vi "Lockin.vi"   [LabVIEW 2019, in "Instrument.Lockin.lvlib"]
uses:
  Instrument.Lockin.lvlib
  Instrument.Lockin/Instrument.Lockin.AppLauncher.vi
  Instrument.Lockin/Instrument.Lockin.lvclass
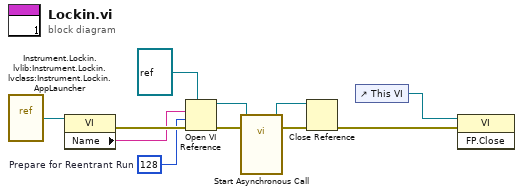
[diagram p0: block diagram]
diagram:
  w3 = 128  # Prepare for Reentrant Run
  n1 = vi-ref "Instrument.Lockin.lvlib:Instrument.Lockin.lvclass:Instrument.Lockin.AppLauncher.vi"() -> (w9:refnum<vi>)
  n2 = property class="VI"(reference=w9) -> (error out=w11:errorcluster, "Name"=w10:string)  [unwired: 1 in, 1 out]
  n3 = Open VI Reference(type specifier VI Refnum (for type only)=refnum<vi> refnum ("reference out"), vi path=w10, options=w3, error in (no error)=w11) -> (vi reference=w8:refnum<vi>, error out=w6:errorcluster)  [unwired: 1 in, 1 out]
  n4 = call-by-ref "Start Asynchronous Call"(reference=w8, error in=w6) -> (reference out=w5:refnum<vi>, error out=w4:errorcluster)  [unwired: 12 in]
  n5 = Close Reference(reference=w5, error in (no error)=w4) -> (error out=w1:errorcluster)
  n6 = control-ref of="This VI"() -> (w2:refnum<vi>)
  n7 = invoke class="VI" method="FP.Close"(reference=w2, error in=w1) -> ()  [unwired: 1 in, 3 out]
